vi "subLoadCommandlineArgs.vi"(11 "Options in":T1={"Path"=path "C:/DependencyInspector/src", "Preview?"=FALSE, "Quiet?"=FALSE, "Show help?"=FALSE}) -> (1 "From command line?":bool, 3 "Options":T1={"Path"=path "C:/DependencyInspector/src", "Preview?"=FALSE, "Quiet?"=FALSE, "Show help?"=FALSE})   [LabVIEW 2020, in "SolutionBuilder.lvlib"]
uses:
  SolutionBuilder.lvlib
  Options.ctl
  <vilib>/regexp/Match Regular Expression.xnode
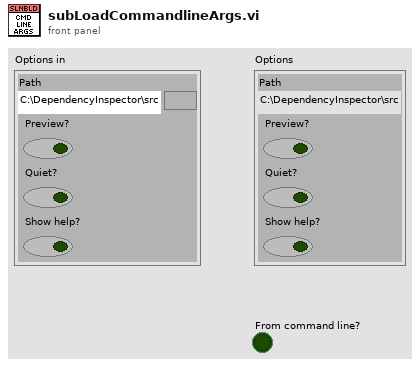
[diagram p1: front panel]
types:
  T1 = typedef "SolutionBuilder.lvlib/Options.ctl" = cluster{"Path":path, "Preview?":bool, "Quiet?":bool, "Show help?":bool}
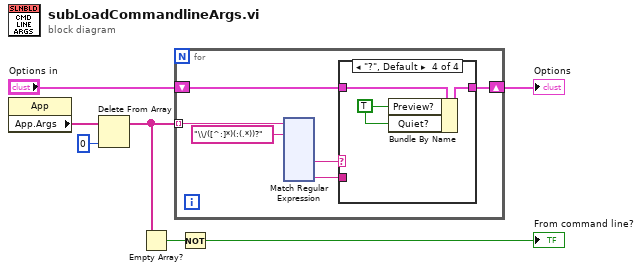
[diagram p0: block diagram]
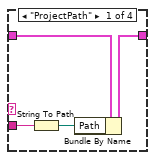
[diagram p2: hidden frame]
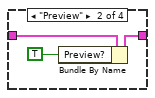
[diagram p3: hidden frame]
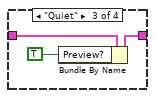
[diagram p4: hidden frame]
diagram:
  n1 = property class="App"() -> ("App.Args"=w6:string[])  [unwired: 2 in, 2 out]
  n2 = Delete From Array(array=w6, index=0) -> (array with subset deleted=w3:string[])  [unwired: 1 in, 1 out]
  n3 = Empty Array?(array=w3) -> (empty?=w2:bool)
  n4 = for {
    tunnel: w3 -> [w13] mode=indexing
    shift-right: [w8] -> w5
    shift-left: "Options in" -> [w11]
    n5 = xnode "Match Regular Expression"("input string"=w13, "regular expression"="\\/([^:]*)(:(.*))?") -> ("submatch 1"=w10:string, "submatch 3"=w9:string)  [unwired: 4 in, 6 out]
    n6 = case shown="\"?\", Default" w10 {
      tunnel: w11 -> [w17 w20 w23 w26]
      tunnel: w9 -> [w15 _ _ _]
      tunnel: [w16 w19 w22 w25] -> w8
      frame "ProjectPath" {
        n7 = String To Path(string=w15) -> (path=w14:path)
        n8 = Bundle By Name(cluster=w17, "Path"=w14) -> (w16:T1)
      }
      frame "Preview" {
        n9 = Bundle By Name(cluster=w20, "Preview?"=TRUE) -> (w19:T1)
      }
      frame "Quiet" {
        n10 = Bundle By Name(cluster=w23, "Preview?"=TRUE) -> (w22:T1)
      }
      frame "?", Default {
        w24 = TRUE ("Preview?")
        n11 = Bundle By Name(cluster=w26, "Preview?"=w24, "Quiet?"=w24) -> (w25:T1)
      }
    }
  }
  "Options" <- w5
  n12 = Not(x=w2) -> (.not. x?=→"From command line?":bool)
